vi "Stop Axis.vi"(4 "error in (no error)":errorcluster, 6 "Axis In":i16, 7 "Controller Reference In":refnum<k7>) -> (0 "error out":errorcluster, 2 "Axis Out":i16, 3 "Controller Reference out":refnum<k7>)   [LabVIEW 2015]
doc: "Stops the movement of the input Axis. The axis is still allowed to decellerate according to it's setup parameters. It will NOT stop the axis movement imediately."
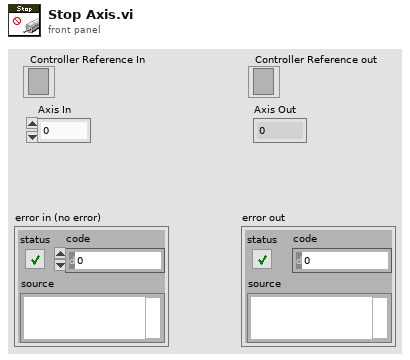
[diagram p1: front panel]
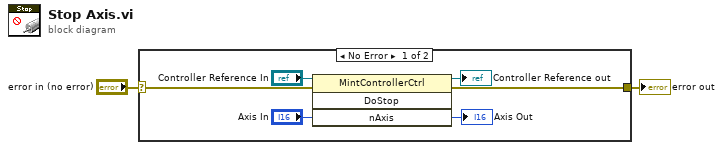
[diagram p0: block diagram]
diagram:
  n1 = case shown="No Error" "error in (no error)" {
    selector: "error in (no error)" -> [w3 w9]
    tunnel: [w6 w9] -> w2
    frame No Error {
      n2 = invoke class="MintControllerCtrl" method="DoStop"(reference="Controller Reference In", error in=w3, "nAxis"="Axis In") -> (reference out=→"Controller Reference out":refnum<k7>, error out=w6:errorcluster, "nAxis"=→"Axis Out":i16)  [unwired: 1 in, 1 out]
    }
    frame Error {
    }
  }
  "error out" <- w2
